vi "Rd Wr settings json Arduino Focus.vi"(8 "error in (no error)":errorcluster, 9 "Settings File":string="CC System Settings.json", 10 "Write? (F:Read)":bool, 11 "Arduino Focus Settings":T1={"Port"="ArduinoFocus", "Homing Parameters"={"Direction"=TRUE, "NUMBER OF  STEPS"=1000, "SPEED STEPS/SEC"=100, "ACC/DECEL STEPS/SEC^2"=100, "EN/DIS?"=TRUE}, "Positions"=[0, 0], "Homed"=[FALSE, FALSE]} {"Homing Parameters"."ACC/DECEL STEPS/SEC^2" max=4000; "Homing Parameters"."SPEED STEPS/SEC" min=20 max=4000 step=10}) -> (0 "error out":errorcluster, 3 "Arduino Focus Settings":T1={"Port"="", "Homing Parameters"={"Direction"=TRUE, "NUMBER OF  STEPS"=13000, "SPEED STEPS/SEC"=1000, "ACC/DECEL STEPS/SEC^2"=1000, "EN/DIS?"=TRUE}, "Positions"=[], "Homed"=[]} {"Homing Parameters"."ACC/DECEL STEPS/SEC^2" max=4000; "Homing Parameters"."SPEED STEPS/SEC" min=20 max=4000 step=10})   [LabVIEW 2024, in "ArduinoFocus.lvclass"]
uses:
  ArduinoFocus.lvclass
  Arduino Focus cluster Settings.ctl
  Motor Control Driver/arduino Motor Control cluster Command.ctl
  2e80df6d-94aa-46b9-8b94-ceea8c057880.vi
  659fb017-0e9f-42f9-b06e-930303f00cbc.vi
  <vilib>/JDP Science/JSONtext/Find Item.vi
  <vilib>/JDP Science/JSONtext/Next JSON Value.vi
  <vilib>/JDP Science/JSONtext/String Subset.vi
  <vilib>/JDP Science/JSONtext/Parsing/Advance past next JSON Value (inlined COPY).vi
  <vilib>/JDP Science/JSONtext/Parsing/Advance past whitespace.vi
  <vilib>/JDP Science/JSONtext/Parsing/Advance past String.vi
  <vilib>/JDP Science/JSONtext/Parsing/Advance past Number.vi
  <vilib>/JDP Science/JSONtext/Parsing/Advance past Line Ending.vi
  <vilib>/JDP Science/JSONtext/Parsing/Parse Full Path or Item Name.vi
  <vilib>/JDP Science/JSONtext/Parsing/Advance past Array.vi
  <vilib>/JDP Science/JSONtext/Parsing/Advance past Object.vi
  <vilib>/JDP Science/JSONtext/support/Error Cluster From Code.vi
  <vilib>/JDP Science/JSONtext/Offset/Find Item Locations by Path.vi
  <vilib>/JDP Science/JSONtext/JSON text to Variant.vi
  <vilib>/JDP Science/JSONtext/Variant to JSON Text.vi
  <vilib>/JDP Science/JSONtext/Set Item.vi
  <vilib>/JDP Science/JSONtext/LVClass Serializer/JSONtext LVClass Serializer.lvclass
  <vilib>/JDP Science/JSONtext/JSONtext.lvlib
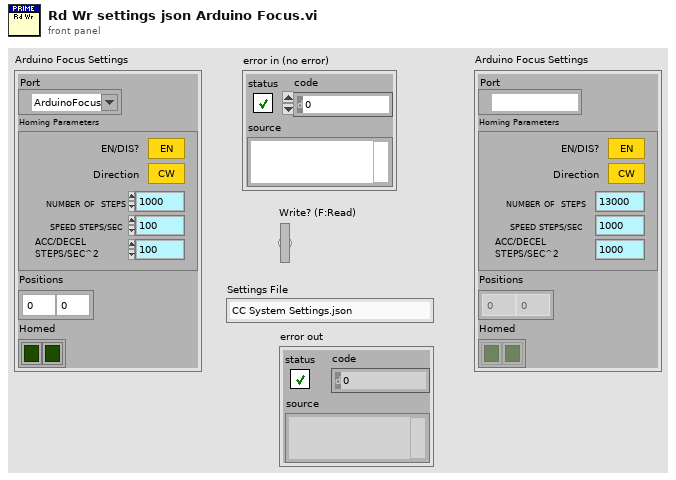
[diagram p1: front panel]
types:
  T1 = typedef "ArduinoFocus.lvclass/Arduino Focus cluster Settings.ctl" = cluster{"Port":refnum<visa-resource-name>, "Homing Parameters":T2, "Positions":i32[], "Homed":bool[]}
  T2 = typedef "arduino Motor Control cluster Command.ctl" = cluster{"Direction":bool, "NUMBER OF  STEPS":u32, "SPEED STEPS/SEC":u16, "ACC/DECEL STEPS/SEC^2":u16, "EN/DIS?":bool}
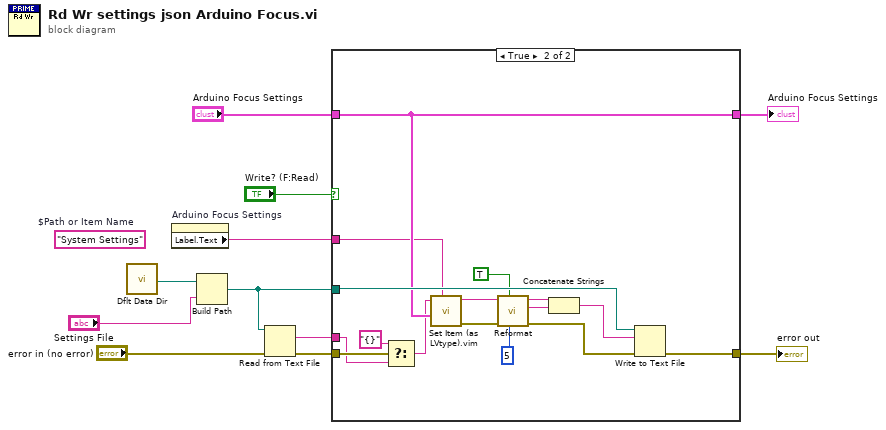
[diagram p0: block diagram]
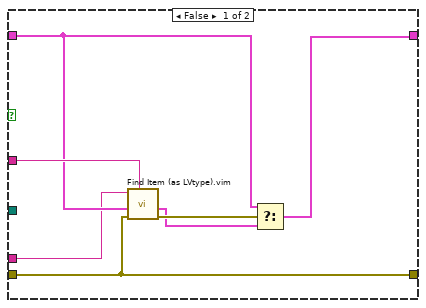
[diagram p2: hidden frame]
diagram:
  (unwired) "System Settings"  # $Path or Item Name
  n1 = call <vilib>:"Dflt Data Dir.vi"() -> ("App:Default Data Directory"=w8:path)
  n2 = property on="Arduino Focus Settings" class="Clust (strict)"() -> ("Label.Text"=w1:string)  [unwired: 2 in, 2 out]
  n3 = Build Path(base path=w8, name or relative path="Settings File") -> (appended path=w2:path)
  n4 = Read from Text File(file (use dialog)=w2, error in="error in (no error)") -> (text=w3:string, error out=w4:errorcluster)  [unwired: 2 in, 2 out]
  n5 = case shown="True" "Write? (F:Read)" {
    tunnel: w4 -> [w12 w30]
    tunnel: "Arduino Focus Settings" -> [w16 w32]
    tunnel: w2 -> [_ w34]
    tunnel: [w12 w33] -> w7
    tunnel: [w18 w32] -> w6
    tunnel: w1 -> [w17 w31]
    tunnel: w3 -> [w13 w28]
    frame False {
      n6 = call "Find Item (as LVtype).vim"("$Path or Item Name"=w17, "error in (no error)"=w12, "Data Type and Default Value"=w16, "JSON"=w13) -> ("error out"=w15:errorcluster, "Data"=w14:T1)  [unwired: 4 in, 2 out]
      n7 = Select(t=w16, s=w15, f=w14) -> (s? t:f=w18:T1)
    }
    frame True {
      n8 = Select(t="{}" ("JSON"), s=w30, f=w28) -> (s? t:f=w27:string)
      n9 = call "Set Item (as LVtype).vim"("$Path or Item Name"=w31, "Anything"=w32, "JSON"=w27) -> ("error out"=w23:errorcluster, "<JSON>"=w24:string)  [unwired: 5 in, 1 out]
      n10 = call <vilib>:"Reformat.vi"("Pretty Print Levels"=5, "Alphabetically Sort Objects"=TRUE, "error in (no error)"=w23, "JSON"=w24) -> ("error out"=w22:errorcluster, "Rest of Input String"=w20:string, "<JSON>"=w21:string)  [unwired: 4 in, 1 out]
      n11 = Concatenate Strings(w21, w20) -> (w19:string)
      n12 = Write to Text File(file (use dialog)=w34, text=w19, error in=w22) -> (error out=w33:errorcluster)  [unwired: 1 in, 2 out]
    }
  }
  "error out" <- w7
  "Arduino Focus Settings" <- w6
